vi "GenerateCLZIssuesMap.vi"(8 "error in (no error)":errorcluster, 11 "CLZ Issues map in":T1(c390)) -> (0 "error out":errorcluster, 3 "CLZ Issues map out":T1(c390))   [LabVIEW 2024]
uses:
  <vilib>/Utility/file.llb/Read Delimited Spreadsheet (string).vi
  <userlib>/_OpenG.lib/string/string.llb/openg_string.lvlib
panel:
  out "all rows":string[][](array[string])
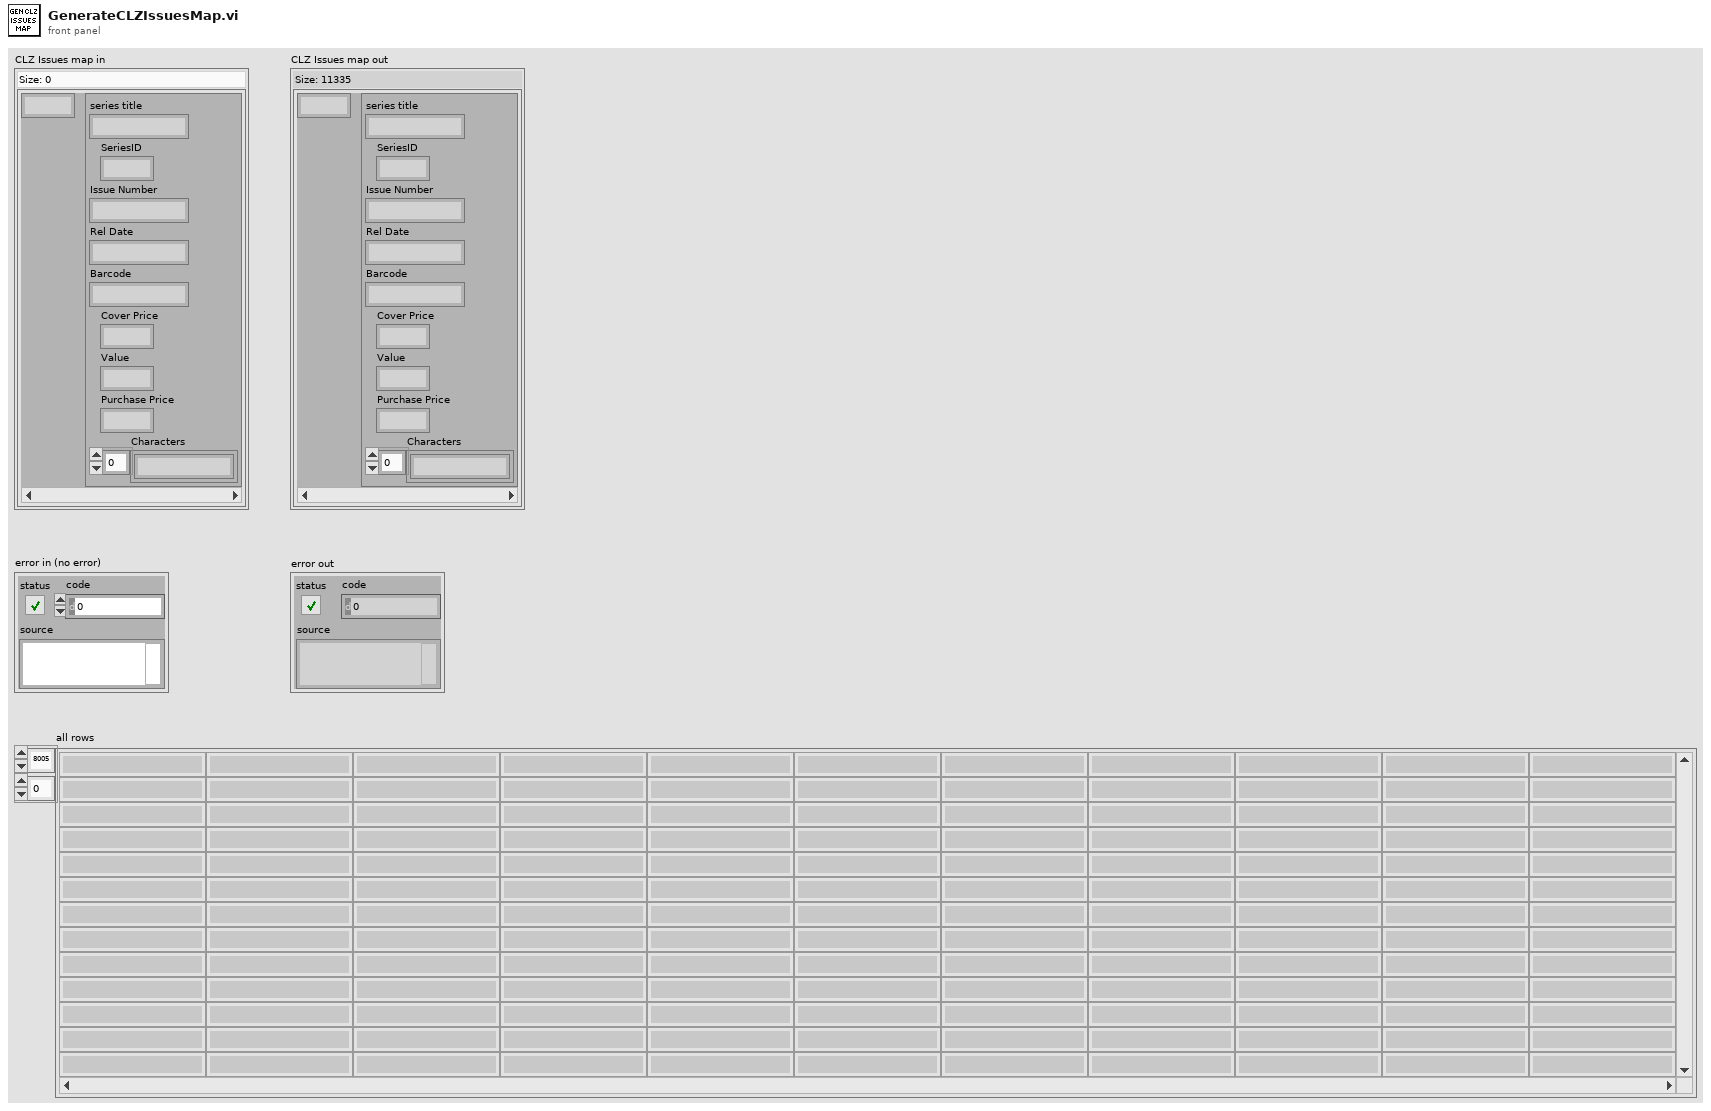
[diagram p1: front panel]
types:
  T1 = map{i32, cluster{"series title":string, "SeriesID":i32, "Issue Number":string, "Rel Date":string, "Barcode":string, "Cover Price":dbl, "Value":dbl, "Purchase Price":dbl, "Characters":string[]}}
  T2 = cluster{"series title":string, "SeriesID":i32, "Issue Number":string, "Rel Date":string, "Barcode":string, "Cover Price":dbl, "Value":dbl, "Purchase Price":dbl, "Characters":string[]}
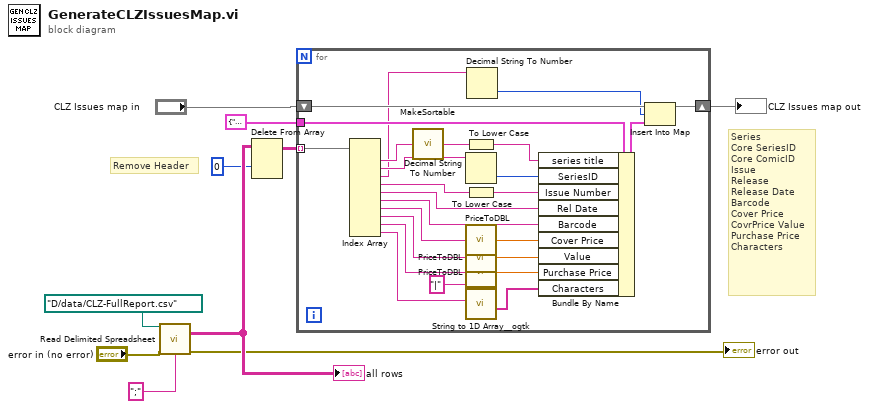
[diagram p0: block diagram]
diagram:
  # "Remove Header"
  # "Series\nCore SeriesID\nCore ComicID\nIssue\nRelease\nRelease Date\nBarcode\nCover Price\nCovrPrice Value\nPurchase Price\nCharacters"
  n1 = call-poly <vilib>:"Read Delimited Spreadsheet.vi"("file path (dialog if empty)"=path "D:/data/CLZ-FullReport.csv", "error in (no error)"="error in (no error)", "delimiter (\\t)"=";" ("delimiter (\\t)")) -> ("all rows"=w8:string[][], "error out"=→"error out":errorcluster)  [unwired: 7 in, 4 out]
  "all rows" <- w8
  n2 = Delete From Array(array=w8, index (row)=0) -> (array with subset deleted=w6:string[][])  [unwired: 2 in, 1 out]
  n3 = for {
    tunnel: w6 -> [w35] mode=indexing
    shift-right: [w34] -> w5
    shift-left: "CLZ Issues map in" -> [w31]
    tunnel: T2 {"series title"="", "SeriesID"=0, "Issue Number"="", "Rel Date"="", "Barcode"="", "Cover Price"=0.0, "Value"=0.0, "Purchase Price"=0.0, "Characters"=[]} -> [w33]
    n4 = Index Array(array=w35) -> (element #1=w30:string, element #2=w27:string, element #3=w25:string, element #4=w24:string, element #5=w22:string, element #6=w21:string, element #7=w20:string, element #8=w17:string, element #9=w16:string, element #10=w13:string)  [unwired: 10 in]
    n5 = call "MakeSortable.vi"("string in"=w30) -> ("string out"=w29:string)
    n6 = To Lower Case(string=w29) -> (all lower case string=w28:string)
    n7 = Decimal String To Number(string=w27) -> (number=w26:i32)  [unwired: 2 in, 1 out]
    n8 = To Lower Case(string=w24) -> (all lower case string=w23:string)
    n9 = call "PriceToDBL.vi"("float string"=w20) -> ("float out"=w19:dbl)
    n10 = call "PriceToDBL.vi"("float string"=w17) -> ("float out"=w18:dbl)
    n11 = call "PriceToDBL.vi"("float string"=w16) -> ("float out"=w15:dbl)
    n12 = call <userlib>:"String to 1D Array__ogtk.vi"("delimiter (Tab)"="|", "string"=w13) -> ("Array of Strings"=w11:string[])  [unwired: 9 in]
    n13 = Decimal String To Number(string=w25) -> (number=w14:i32)  [unwired: 2 in, 1 out]
    n14 = Bundle By Name(cluster=w33, "series title"=w28, "SeriesID"=w26, "Issue Number"=w23, "Rel Date"=w22, "Barcode"=w21, "Cover Price"=w19, "Value"=w18, "Purchase Price"=w15, "Characters"=w11) -> (w32:T2)
    n15 = Insert Into Map(map in=w31, key=w14, value=w32) -> (map out=w34:T1)  [unwired: 2 out]
  }
  "CLZ Issues map out" <- w5
